vi "TestHorizontalLineto.vi"(8 "error in (no error)":errorcluster) -> (0 "error out":errorcluster)   [LabVIEW 2019]
uses:
  PathCommands.LineTo/PathCommands.LineTo.lvclass
  <vilib>/addons/_JKI Toolkits/Caraya/classes/Assert/Assert Equal Value_Variant.vi
  <vilib>/addons/_JKI Toolkits/Caraya/classes/Assert/Assert False.vi
  <vilib>/addons/_JKI Toolkits/Caraya/classes/Assert/Assert True.vi
  <vilib>/addons/_JKI Toolkits/Caraya/classes/Assert/Assert.lvclass
  <vilib>/addons/_JKI Toolkits/Caraya/classes/Test/Test.lvclass
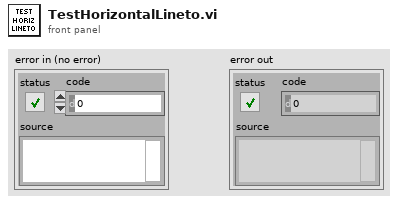
[diagram p1: front panel]
types:
  T1 = enum16{"None", "After", "Before", "Last", "First"}[]
  T2 = typedef "PathCommands.lvclass/Point.ctl" = cluster{"X":dbl, "Y":dbl}
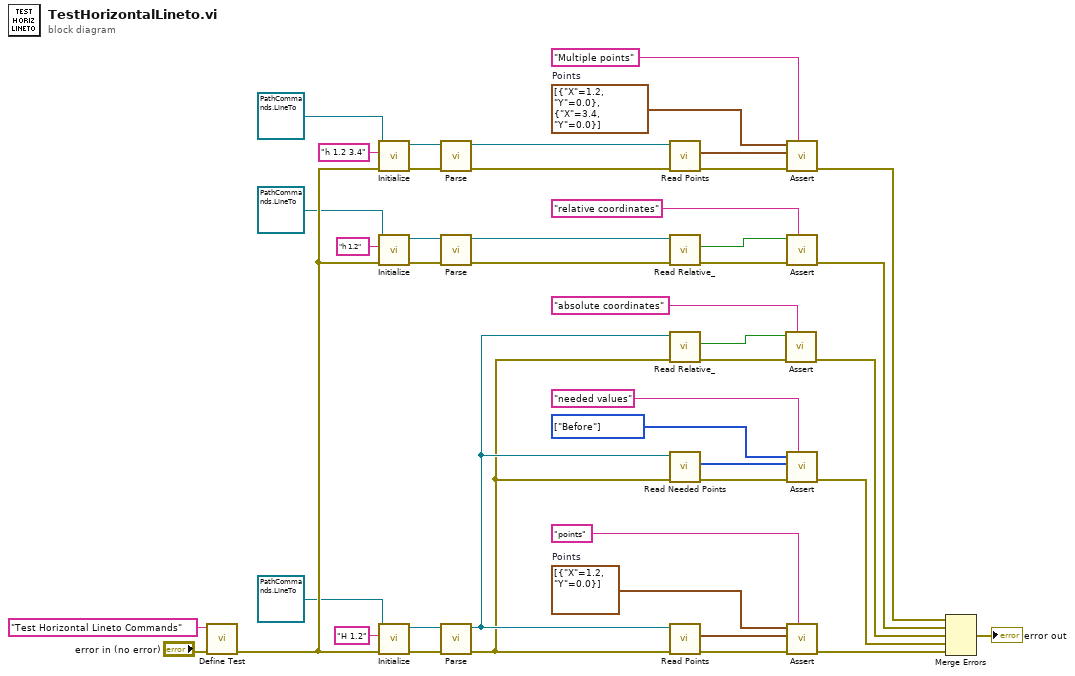
[diagram p0: block diagram]
diagram:
  w10 = cluster{"X":dbl, "Y":dbl}[] [{"X"=1.2, "Y"=0.0}, {"X"=3.4, "Y"=0.0}]  # Points
  w38 = T1 [enum."Before"] items=["None", "After", "Before", "Last", "First"] ("Needed Points 4")
  w35 = cluster{"X":dbl, "Y":dbl}[] [{"X"=1.2, "Y"=0.0}]  # Points
  n1 = call <vilib>:"Define Test.vi"("error in (no error)"="error in (no error)", "Label (VI Title)"="Test Horizontal Lineto Commands") -> ("error out"=w14:errorcluster)  [unwired: 8 in, 1 out]
  n2 = call-dynamic "Initialize.vi"("error in (no error)"=w14, "CommandText"="h 1.2 3.4", "PathCommands.LineTo in"=refnum<class "PathCommands.LineTo.lvclass"> refnum) -> ("error out"=w15:errorcluster, "PathCommands.LineTo out"=w17:refnum<class "PathCommands.LineTo.lvclass">)  [unwired: 7 in]
  n3 = call-dynamic "Initialize.vi"("error in (no error)"=w14, "CommandText"="h 1.2", "PathCommands.LineTo in"=refnum<class "PathCommands.LineTo.lvclass"> refnum) -> ("error out"=w25:errorcluster, "PathCommands.LineTo out"=w23:refnum<class "PathCommands.LineTo.lvclass">)  [unwired: 7 in]
  n4 = call-dynamic "Initialize.vi"("error in (no error)"=w14, "CommandText"="H 1.2", "PathCommands.LineTo in"=refnum<class "PathCommands.LineTo.lvclass"> refnum) -> ("error out"=w43:errorcluster, "PathCommands.LineTo out"=w45:refnum<class "PathCommands.LineTo.lvclass">)  [unwired: 7 in]
  n5 = call-dynamic "Parse.vi"("error in (no error)"=w15, "PathCommands.LineTo in"=w17) -> ("error out"=w8:errorcluster, "PathCommands.LineTo out"=w9:refnum<class "PathCommands.LineTo.lvclass">)  [unwired: 8 in]
  n6 = call-dynamic "Parse.vi"("error in (no error)"=w25, "PathCommands.LineTo in"=w23) -> ("error out"=w18:errorcluster, "PathCommands.LineTo out"=w19:refnum<class "PathCommands.LineTo.lvclass">)  [unwired: 8 in]
  n7 = call-dynamic "Parse.vi"("error in (no error)"=w43, "PathCommands.LineTo in"=w45) -> ("error out"=w30:errorcluster, "PathCommands.LineTo out"=w31:refnum<class "PathCommands.LineTo.lvclass">)  [unwired: 8 in]
  n8 = call-dynamic "Read Points.vi"("error in (no error)"=w8, "PathCommands in"=w9) -> ("error out"=w12:errorcluster, "Points"=w11:T2[])  [unwired: 7 in, 1 out]
  n9 = call-dynamic "Read Relative_.vi"("error in (no error)"=w18, "PathCommands in"=w19) -> ("error out"=w21:errorcluster, "Relative?"=w22:bool)  [unwired: 7 in, 1 out]
  n10 = call-dynamic "Read Relative_.vi"("error in (no error)"=w30, "PathCommands in"=w31) -> ("error out"=w41:errorcluster, "Relative?"=w40:bool)  [unwired: 7 in, 1 out]
  n11 = call-dynamic "Read Needed Points.vi"("error in (no error)"=w30, "PathCommands in"=w31) -> ("error out"=w37:errorcluster, "Needed Points"=w36:T1)  [unwired: 7 in, 1 out]
  n12 = call-dynamic "Read Points.vi"("error in (no error)"=w30, "PathCommands in"=w31) -> ("error out"=w33:errorcluster, "Points"=w34:T2[])  [unwired: 7 in, 1 out]
  n13 = call-poly <vilib>:"Assert.vi"("Label"="absolute coordinates", "error in (no error)"=w41, "False?"=w40) -> ("error out"=w3:errorcluster)  [unwired: 7 in, 1 out]
  n14 = call-poly <vilib>:"Assert.vi"("Label"="Multiple points", "error in (no error)"=w12, "Y"=w11, "X"=w10) -> ("error out"=w1:errorcluster)  [unwired: 6 in, 1 out]
  n15 = call-poly <vilib>:"Assert.vi"("Label"="relative coordinates", "error in (no error)"=w21, "True?"=w22) -> ("error out"=w2:errorcluster)  [unwired: 7 in, 1 out]
  n16 = call-poly <vilib>:"Assert.vi"("Label"="needed values", "error in (no error)"=w37, "Y"=w36, "X"=w38) -> ("error out"=w4:errorcluster)  [unwired: 6 in, 1 out]
  n17 = call-poly <vilib>:"Assert.vi"("Label"="points", "error in (no error)"=w33, "Y"=w34, "X"=w35) -> ("error out"=w29:errorcluster)  [unwired: 6 in, 1 out]
  n18 = Merge Errors(w1, w2, w3, w4, w29) -> (→"error out":errorcluster)
